vi "Write singleplayer.vi"(8 "error in (no error)":errorcluster, 10 "singleplayer":bool, 11 "Pong in":refnum<class "Pong.lvclass">) -> (0 "error out":errorcluster, 3 "Pong out":refnum<class "Pong.lvclass">)   [LabVIEW 2019, in "RT_Game.lvlib" / "Pong.lvclass"]
uses:
  Pong.lvclass
  Pong.lvclass/Pong.ctl
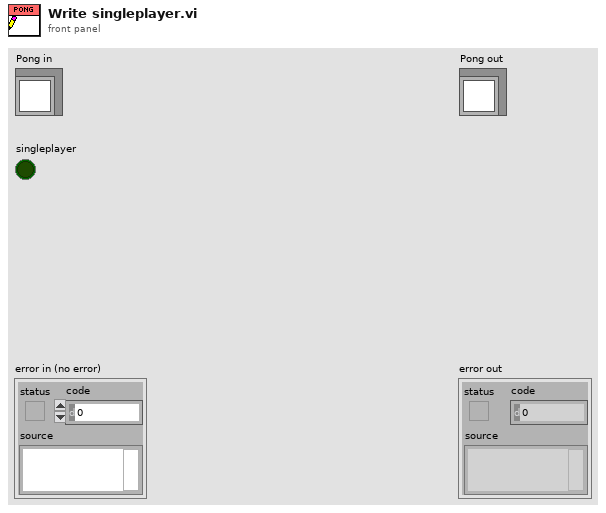
[diagram p1: front panel]
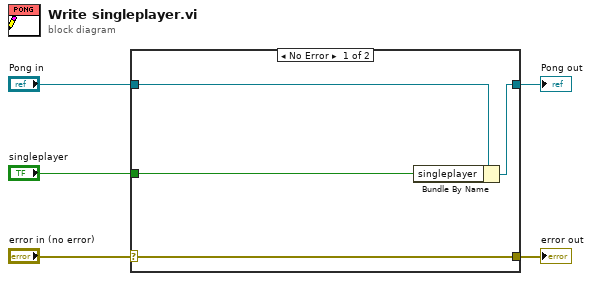
[diagram p0: block diagram]
diagram:
  n1 = case shown="No Error" "error in (no error)" {
    selector: "error in (no error)" -> [w9 w10]
    tunnel: [w9 w10] -> w4
    tunnel: [w7 w11] -> w2
    tunnel: "Pong in" -> [w8 w11]
    tunnel: "singleplayer" -> [w6 _]
    frame No Error {
      n2 = Bundle By Name(cluster=w8, "singleplayer"=w6) -> (w7:refnum<class "Pong.lvclass">)
    }
    frame Error {
    }
  }
  "error out" <- w4
  "Pong out" <- w2
